vi "Acoustic Noise.vi"(0 "TSM context":T2, 1 "Capture Duration (s)":dbl, 5 "Minimum Frequency (Hz)":dbl=20.0 format="%#_13g", 7 "Maximum Frequency(Hz)":dbl=200.0 format="%#_13g", 9 "Window(Rectangle)":T1 items=["Rectangle"=0, "Hanning"=1, "Hamming"=2, "Blackman-Harris"=3, "Exact Blackman"=4, "Blackman"=5, "Flat Top"=6, "4 Term B-Harris "=7, "7 Term B-Harris"=8, "Low Sidelobe"=9, "Blackman Nuttall"=11, "Triangle"=30, "Bartlett-Hanning"=31, "Bohman"=32, "Parzen"=33, "Welch"=34, "Kaiser"=60, "Dolph-Chebyshev"=61, "Gaussian"=62]) -> (4 "Per-Site Waveform Out":waveform(dbl)[](array[waveform]), 15 "error out":errorcluster)   [LabVIEW 2020]
doc: "Acoustic Noise VI help to capture the noise waveform from the reference mic and the DUT, and calculate the A-weighted noise (dBA) for those waveforms"
uses:
  <vilib>/NI_TestStand_SemiconductorModule/NI_TestStand_Semiconductor_Module.lvlibp/PinMap/General/SemiconductorModuleContext.ctl
  <vilib>/Analysis/4window.llb/windowTd.ctl
  <vilib>/NI_TestStand_SemiconductorModule/NI_TestStand_Semiconductor_Module.lvlibp/PinMap/TagProvider/TSM_Pin.ctl
  a997cb1e-d7f5-4ebd-8397-b6f8af7b1bae.vi
  a7360eba-c132-4539-a123-ad9ae009621d.vi
  <vilib>/NI_TestStand_SemiconductorModule/NI_TestStand_Semiconductor_Module.lvlibp/PinMap/General/Publish/PublishDataDoubleFunctionalTest.vi
  <vilib>/NI_TestStand_SemiconductorModule/NI_TestStand_Semiconductor_Module.lvlibp
  <vilib>/Analysis/NI_AALPro.lvlib
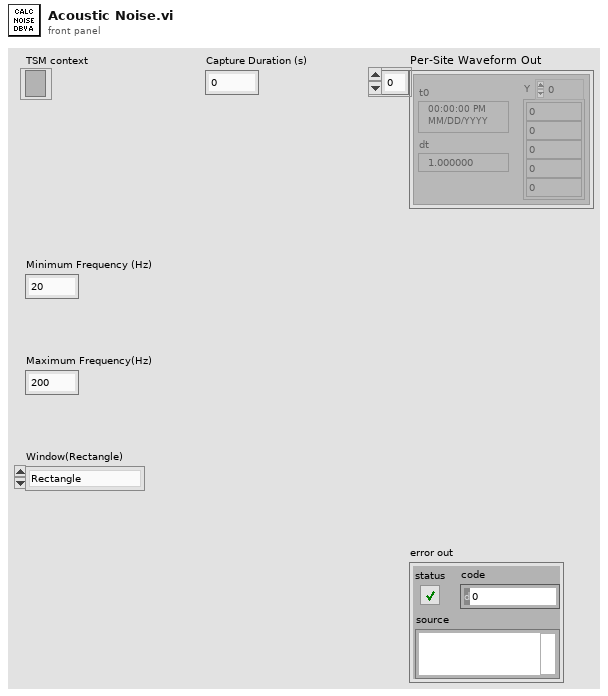
[diagram p1: front panel]
types:
  T1 = typedef "NI_AALPro.lvlib/windowTd.ctl" = u32
  T2 = typedef "NI_TestStand_Semiconductor_Module.lvlibp/SemiconductorModuleContext.ctl" = refnum<k7>
  T3 = typedef "NI_TestStand_Semiconductor_Module.lvlibp/TSM_Pin.ctl" = tag
  T4 = typedef "TSM DAQmx Multi-Task.ctl" = cluster{"Pin Query Context":refnum<class "MultiplePinMultipleSessionQueryContext.lvclass">, "SSC":T5[], "Site Numbers":i32[], "Pins":tag[]}
  T5 = typedef "SSC DAQmx.ctl" = cluster{"DAQmx Task ":refnum<k21>, "Channels":string, "Channel Lists":string}
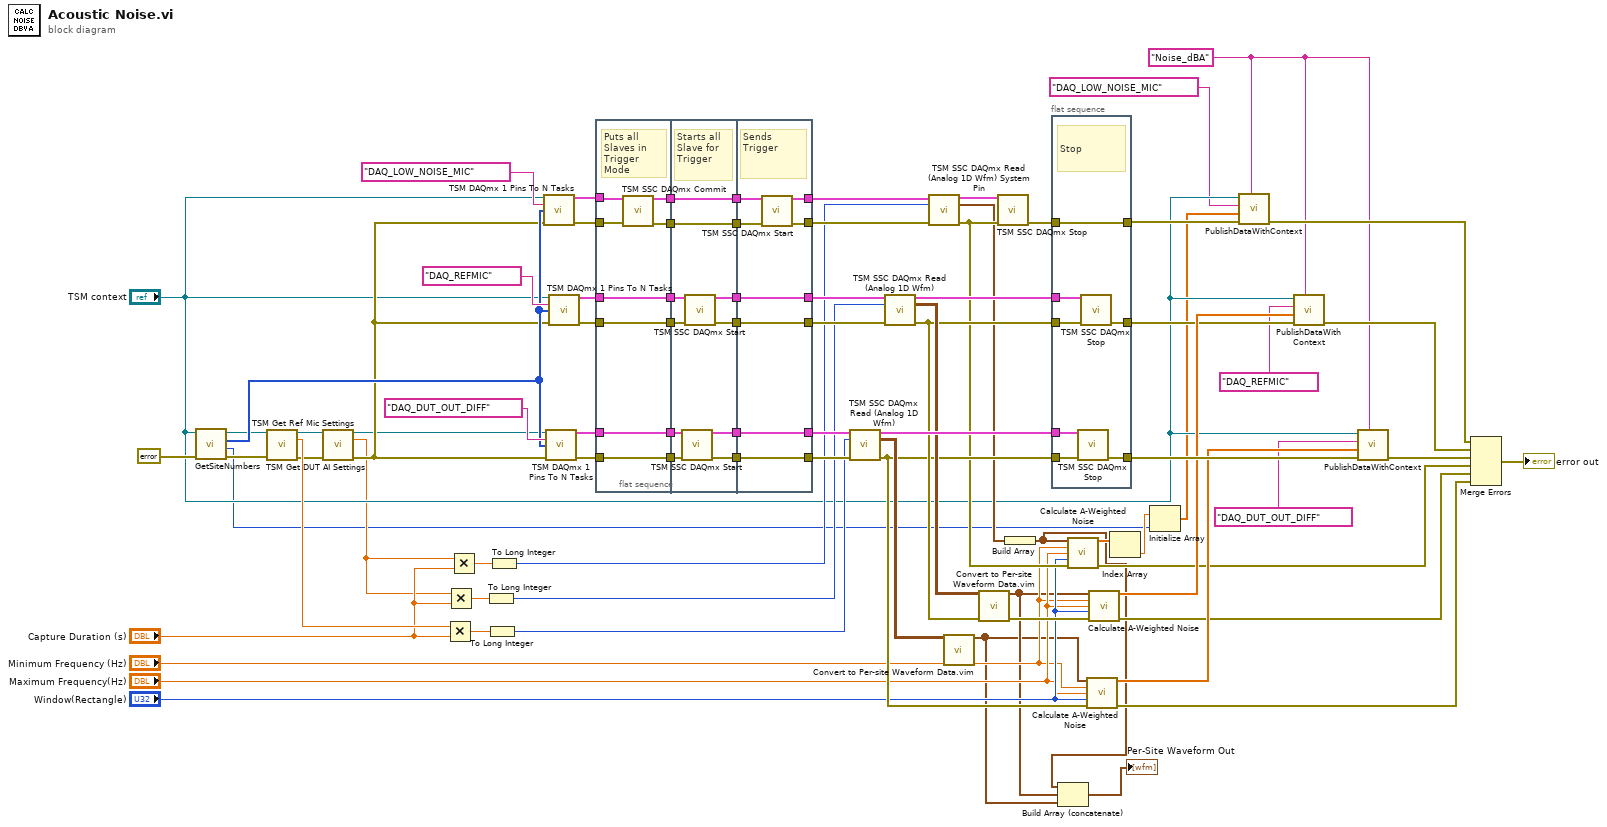
[diagram p0: block diagram]
diagram:
  w7 = "Noise_dBA"
  n1 = call <vilib>:"GetSiteNumbers.vi"("error in (no error)"=errorcluster {"status"=FALSE, "code"=0, "source"=""} ("error in"), "Semiconductor Module Context"="TSM context") -> ("error out"=w30:errorcluster, "Number Of Sites"=w10:i32, "Site Numbers"=w49:i32[], "Semiconductor Module Context Out"=w29:T2)  [unwired: 6 in]
  n2 = call "TSM Get DUT AI Settings.vi"("TSM context"=w29, "error in (no error)"=w30) -> ("TSM context Out"=w57:T2, "Sampling Rate (Hz)"=w60:dbl, "error out"=w58:errorcluster)  [unwired: 9 in, 2 out]
  n3 = call "TSM Get Ref Mic Settings.vi"("TSM context"=w57, "error in (no error)"=w58) -> ("TSM context Out"=w27:T2, "Sampling Rate (Hz)"=w12:dbl, "error out"=w28:errorcluster)  [unwired: 8 in, 3 out]
  n4 = Multiply(x=w60, y="Capture Duration (s)") -> (x*y=w61:dbl)
  n5 = Multiply(x=w12, y="Capture Duration (s)") -> (x*y=w56:dbl)
  n6 = Multiply(x=w12, y="Capture Duration (s)") -> (x*y=w26:dbl)
  n7 = To Long Integer(number=w56) -> (32bit integer=w55:i32)
  n8 = To Long Integer(number=w61) -> (32bit integer=w59:i32)
  n9 = To Long Integer(number=w26) -> (32bit integer=w24:i32)
  n10 = call "TSM DAQmx 1 Pins To N Tasks.vi"("TSM context"="TSM context", "Pins"=tag "DAQ_LOW_NOISE_MIC", "Site Numbers"=w49, "error in"=w28) -> ("DAQ TSM Out"=w43:T4, "error out"=w44:errorcluster)  [unwired: 10 in]
  n11 = call "TSM DAQmx 1 Pins To N Tasks.vi"("TSM context"=w27, "Pins"=tag "DAQ_DUT_OUT_DIFF", "Site Numbers"=w49, "error in"=w28) -> ("DAQ TSM Out"=w78:T4, "error out"=w77:errorcluster)  [unwired: 10 in]
  n12 = call "TSM DAQmx 1 Pins To N Tasks.vi"("TSM context"="TSM context", "Pins"=tag "DAQ_REFMIC", "Site Numbers"=w49, "error in"=w28) -> ("DAQ TSM Out"=w69:T4, "error out"=w70:errorcluster)  [unwired: 10 in]
  n13 = flat-sequence {
    tunnel: w69 -> [w87]
    tunnel: w70 -> [w88]
    tunnel: w77 -> [w89]
    tunnel: w78 -> [w90]
    tunnel: [w90] -> w48
    tunnel: [w89] -> w47
    tunnel: [w88] -> w46
    tunnel: [w87] -> w45
    tunnel: w44 -> [w86]
    tunnel: w43 -> [w85]
    tunnel: [w84] -> w42
    tunnel: [w83] -> w41
    tunnel: w48 -> [w98]
    tunnel: w47 -> [w97]
    tunnel: w46 -> [w96]
    tunnel: w45 -> [w95]
    tunnel: w42 -> [w92]
    tunnel: w41 -> [w91]
    tunnel: [w100] -> w40
    tunnel: [w99] -> w39
    tunnel: [w94] -> w38
    tunnel: [w93] -> w37
    tunnel: [w92] -> w36
    tunnel: [w91] -> w35
    tunnel: [w105] -> w66
    tunnel: [w106] -> w67
    tunnel: [w107] -> w80
    tunnel: [w108] -> w81
    tunnel: w40 -> [w108]
    tunnel: w39 -> [w107]
    tunnel: w38 -> [w106]
    tunnel: w37 -> [w105]
    tunnel: w36 -> [w104]
    tunnel: [w103] -> w33
    tunnel: w35 -> [w102]
    tunnel: [w101] -> w32
    frame #0 {
      # "Puts all Slaves in Trigger Mode"
      n14 = call "TSM SSC DAQmx Commit.vi"("TSM DAQmx In"=w85, "error in (no error)"=w86) -> ("TSM DAQmx Out"=w83:T4, "error out"=w84:errorcluster)  [unwired: 12 in]
    }
    frame #1 {
      # "Starts all Slave for Trigger"
      n15 = call "TSM SSC DAQmx Start.vi"("TSM DAQmx In"=w98, "error in (no error)"=w97) -> ("TSM DAQmx Out"=w99:T4, "error out"=w100:errorcluster)  [unwired: 12 in]
      n16 = call "TSM SSC DAQmx Start.vi"("TSM DAQmx In"=w95, "error in (no error)"=w96) -> ("TSM DAQmx Out"=w94:T4, "error out"=w93:errorcluster)  [unwired: 12 in]
    }
    frame #2 {
      # "Sends Trigger"
      n17 = call "TSM SSC DAQmx Start.vi"("TSM DAQmx In"=w102, "error in (no error)"=w104) -> ("TSM DAQmx Out"=w101:T4, "error out"=w103:errorcluster)  [unwired: 12 in]
    }
  }
  n18 = call "TSM SSC DAQmx Read (Analog 1D Wfm).vi"("DAQ TSM in"=w80, "Samples to read"=w59, "error in"=w81) -> ("DAQ TSM Out"=w79:T4, "Per-Site Per-Pin Waveforms Out"=w76:waveform(dbl)[][], "error out"=w53:errorcluster)  [unwired: 10 in]
  n19 = call "TSM SSC DAQmx Read (Analog 1D Wfm).vi"("DAQ TSM in"=w67, "Samples to read"=w55, "error in"=w66) -> ("DAQ TSM Out"=w68:T4, "Per-Site Per-Pin Waveforms Out"=w71:waveform(dbl)[][], "error out"=w54:errorcluster)  [unwired: 10 in]
  n20 = call "TSM SSC DAQmx Read (Analog 1D Wfm) System Pin.vi"("DAQ TSM in"=w32, "Samples to read"=w24, "error in"=w33) -> ("DAQ TSM Out"=w31:T4, "System-Pin Waveforms Out"=w22:waveform(dbl), "error out"=w23:errorcluster)  [unwired: 10 in]
  n21 = call "Convert to Per-site Waveform Data.vim"("Per-Site Per-Pin Waveform In"=w76) -> ("Per-Site Waveform Out"=w2:waveform(dbl)[])  [unwired: 14 in]
  n22 = call "Convert to Per-site Waveform Data.vim"("Per-Site Per-Pin Waveform In"=w71) -> ("Per-Site Waveform Out"=w3:waveform(dbl)[])  [unwired: 14 in]
  n23 = call "TSM SSC DAQmx Stop.vi"("TSM DAQmx In"=w31, "error in (no error)"=w23) -> ("error out"=w34:errorcluster)  [unwired: 12 in, 1 out]
  n24 = Build Array(w22) -> (w4:waveform(dbl)[])
  n25 = flat-sequence {
    tunnel: w79 -> [w115]
    tunnel: [w114] -> w75
    tunnel: [w113] -> w72
    tunnel: w68 -> [w112]
    tunnel: w54 -> [w111]
    tunnel: w53 -> [w110]
    tunnel: w34 -> [w109]
    tunnel: [w109] -> w16
    frame #0 {
      # "Stop"
      n26 = call "TSM SSC DAQmx Stop.vi"("TSM DAQmx In"=w115, "error in (no error)"=w110) -> ("error out"=w114:errorcluster)  [unwired: 12 in, 1 out]
      n27 = call "TSM SSC DAQmx Stop.vi"("TSM DAQmx In"=w112, "error in (no error)"=w111) -> ("error out"=w113:errorcluster)  [unwired: 12 in, 1 out]
    }
  }
  n28 = Build Array (concatenate)(w4, w3, w2) -> (→"Per-Site Waveform Out":waveform(dbl)[])
  n29 = call "Calculate A-Weighted Noise.vi"("Waveform in"=w4, "fmin (Hz)"="Minimum Frequency (Hz)", "fmax (Hz)"="Maximum Frequency(Hz)", "Window(Rectangle)"="Window(Rectangle)", "error in"=w23) -> ("Noise (dB A-weighted)"=w13:dbl[], "error out"=w17:errorcluster)  [unwired: 9 in]
  n30 = call "Calculate A-Weighted Noise.vi"("Waveform in"=w2, "fmin (Hz)"="Minimum Frequency (Hz)", "fmax (Hz)"="Maximum Frequency(Hz)", "Window(Rectangle)"="Window(Rectangle)", "error in"=w53) -> ("Noise (dB A-weighted)"=w74:dbl[], "error out"=w51:errorcluster)  [unwired: 9 in]
  n31 = call "Calculate A-Weighted Noise.vi"("Waveform in"=w3, "fmin (Hz)"="Minimum Frequency (Hz)", "fmax (Hz)"="Maximum Frequency(Hz)", "Window(Rectangle)"="Window(Rectangle)", "error in"=w54) -> ("Noise (dB A-weighted)"=w73:dbl[], "error out"=w18:errorcluster)  [unwired: 9 in]
  n32 = Index Array(array=w13) -> (element=w11:dbl)  [unwired: 1 in]
  n33 = Initialize Array(w11, w10) -> (w9:dbl[])
  n34 = call-poly <vilib>:"PublishDataWithContext.vi"("Published Data Id"=w7, "error in (no error)"=w16, "Data In"=w9, "Pin"=T3 "DAQ_LOW_NOISE_MIC", "Semiconductor Module Context"="TSM context") -> ("error out"=w15:errorcluster)  [unwired: 5 in, 1 out]
  n35 = call-poly <vilib>:"PublishDataWithContext.vi"("Published Data Id"=w7, "error in (no error)"=w72, "Data In"=w73, "Pin"=T3 "DAQ_REFMIC", "Semiconductor Module Context"="TSM context") -> ("error out"=w64:errorcluster)  [unwired: 5 in, 1 out]
  n36 = call-poly <vilib>:"PublishDataWithContext.vi"("Published Data Id"=w7, "error in (no error)"=w75, "Data In"=w74, "Pin"=T3 "DAQ_DUT_OUT_DIFF", "Semiconductor Module Context"="TSM context") -> ("error out"=w52:errorcluster)  [unwired: 5 in, 1 out]
  n37 = Merge Errors(w15, w64, w52, w17, w18, w51) -> (→"error out":errorcluster)
